vi "lockin - zero amplitude.vi"(8 "error in (no error)":errorcluster, 10 "measure\noffset?":bool, 11 "Instrument.DAQ":refnum<class "Instrument.DAQ.lvclass">) -> (0 "error out":errorcluster, 3 "Instrument.DAQ out":refnum<class "Instrument.DAQ.lvclass">)   [LabVIEW 2019, in "Instrument.DAQ.lvclass"]
uses:
  Instrument.DAQ.lvclass
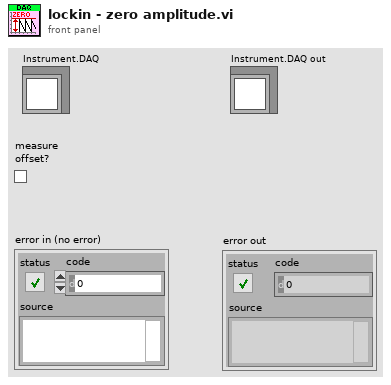
[diagram p1: front panel]
types:
  T1 = typedef "Instrument.DAQ.lvclass/AO.Channel--Cluster--Array.ctl" = T2[]
  T2 = typedef "Instrument.DAQ.lvclass/AO.Channel--Cluster.ctl" = cluster{"Enable?":bool, "Channel":i32, "Amplitude":dbl, "Offset":dbl, "Frequency":dbl, "Phase":dbl, "Function":T3, "Sweeping?":bool}
  T3 = typedef "Instrument.DAQ.lvclass/AO.Channel.Function--Enum.ctl" = enum16{"Sine", "Triangle", "Square"}
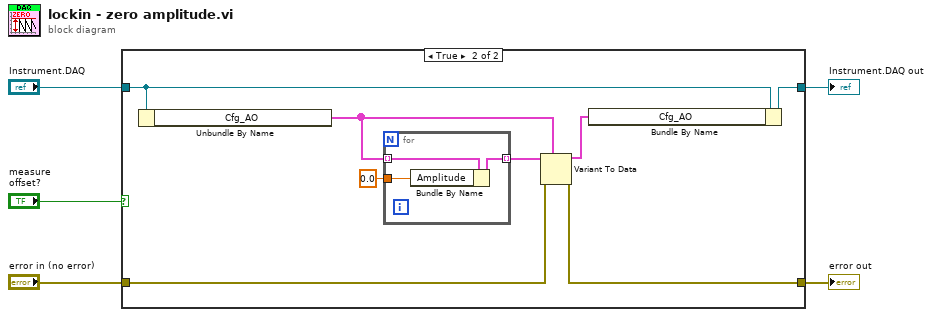
[diagram p0: block diagram]
diagram:
  n1 = case shown="True" "measure\noffset?" {
    tunnel: "Instrument.DAQ" -> [w7 w15]
    tunnel: [w7 w13] -> w4
    tunnel: "error in (no error)" -> [w6 w11]
    tunnel: [w6 w10] -> w1
    frame False {
    }
    frame True {
      n2 = Unbundle By Name(w15) -> ("Cfg_AO"=w8:T1)
      n3 = for {
        tunnel: w8 -> [w17] mode=indexing
        tunnel: 0.0 ("element") -> [w18]
        tunnel: [w16] -> w12 mode=indexing
        n4 = Bundle By Name(cluster=w17, "Amplitude"=w18) -> (w16:T2)
      }
      n5 = Variant To Data(error in=w11, type=w8, Variant=w12) -> (data=w9:T1, error out=w10:errorcluster)
      n6 = Bundle By Name(cluster=w15, "Cfg_AO"=w9) -> (w13:refnum<class "Instrument.DAQ.lvclass">)
    }
  }
  "Instrument.DAQ out" <- w4
  "error out" <- w1
